vi "初始化报警记录清单.vi"   [LabVIEW 2013]
types:
  T1 = enum16{"open", "replace", "create", "open or create", "replace or create", "replace or create with confirmation"}
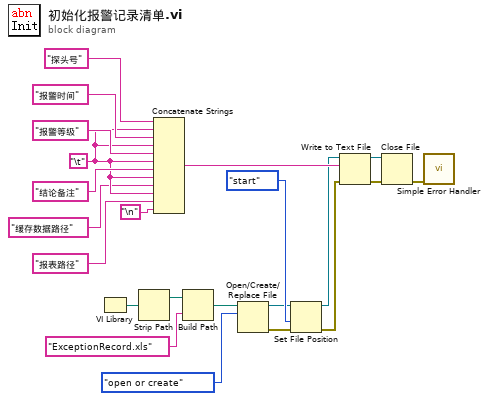
[diagram p0: block diagram]
diagram:
  w4 = "\t"
  n1 = VI Library() -> (path=w11:path)
  n2 = Strip Path(path=w11) -> (stripped path=w10:path)  [unwired: 1 out]
  n3 = Concatenate Strings("探头号", w4, "报警时间", w4, "报警等级", w4, "结论备注", w4, "缓存数据路径" ("字符串"), w4, "报表路径" ("字符串"), "\n") -> (w17:string)
  n4 = Build Path(base path=w10, name or relative path="ExceptionRecord.xls" ("保存文件名")) -> (appended path=w9:path)
  n5 = Open/Create/Replace File(file path (use dialog)=w9, operation (0:open)=T1."open or create" ("操作(0:open)")) -> (refnum out=w12:refnum<file>, error out=w13:errorcluster)  [unwired: 1 in, 4 out]
  n6 = Set File Position(refnum=w12, from (0:start)=enum16{"start", "end", "current"}."start" ("自（0:起始）"), error in=w13) -> (refnum out=w14:refnum<file>, error out=w15:errorcluster)  [unwired: 1 out]
  n7 = Write to Text File(file (use dialog)=w14, text=w17, error in=w15) -> (refnum out=w6:refnum<file>, error out=w5:errorcluster)  [unwired: 2 out]
  n8 = Close File(refnum=w6, error in=w5) -> (error out=w7:errorcluster)  [unwired: 1 out]
  n9 = call <vilib>:"Simple Error Handler.vi"("error in (no error)"=w7) -> ()  [unwired: 1 in, 8 out]
